vi "Power Of X.vi"   [LabVIEW 2018, in "NI_Matrix.lvlib"]
doc: "Computes the nth power of the input matrix."
uses:
  NI_Matrix.lvlib
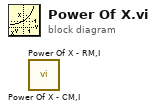
[diagram p0: block diagram]
diagram:
  n1 = call "Power Of X - CM,I.vi"() -> ()  [unwired: 2 in, 1 out]
  n2 = call "Power Of X - RM,I.vi"() -> ()  [unwired: 2 in, 1 out]
